vi "Calling or Specified VI's Clustered Controls Details, rev a.vi"(0 "Call heirarchy index\n(1 = calling VI, \n2 = its calling VI), etc)":i32=2, 11 "error in (no error)":errorcluster) -> (1 "Direct-access\ncontrols for\nrelabeling":refnum<vi>[](array[refnum]), 2 "Refs to controls on panel":refnum<vi>[](array[refnum]), 3 "Direct-access\ncontrols for\nrelabeling: captions":string[](array[string])=["Application Directory", "Direct Name 1", "Direct Position 1", "Direct Jog - 1", "Direct Jog + 1", "Direct Step (mm) 1", "Direct Halt Axis 1", "Direct Settings 1", "Direct Moving 1", "Direct New target 1", "Direct OK 1", "Direct Home Axis 1", "Direct Home Axis 2", "Direct OK 2", "Direct New target 2", "Direct Moving 2", "Direct Settings 2", "Direct Halt Axis 2", "Direct Step (mm) 2", "Direct Jog + 2", "Direct Jog - 2", "Direct Position 2", "Direct Name 2", "Direct Home Axis 3", "Direct OK 3", "Direct New target 3", "Direct Moving 3", "Direct Settings 3", "Direct Halt Axis 3", "Direct Step (mm) 3", "Direct Jog + 3", "Direct Jog - 3", "Direct Position 3", "Direct Name 3", "Direct Home Axis 4", "Direct OK 4", "Direct New target 4", "Direct Moving 4", "Direct Settings 4", "Direct Halt Axis 4", "Direct Step (mm) 4", "Direct Jog + 4", "Direct Jog - 4", "Direct Position 4", "Direct Name 4", "Direct Home Axis 5", "Direct OK 5", "Direct New target 5", "Direct Moving 5", "Direct Settings 5", "Direct Halt Axis 5", "Direct Step (mm) 5", "Direct Jog + 5", "Direct Jog - 5", "Direct Position 5", "Direct Name 5", "Direct Home Axis 6", "Direct OK 6", "Direct New target 6", "Direct Moving 6", "Direct Settings 6", "Direct Halt Axis 6", "Direct Step (mm) 6", "Direct Jog + 6", "Direct Jog - 6", "Direct Position 6", "Direct Name 6"], 4 "Names of Clusters":string[](array[string])=["error out"], 6 "Controls in\nthose clusters":string[][](array[string])=[["status", "code", "source"]], 10 "Refs to clusters":refnum<vi>[](array[refnum]), 12 "Controls directly on tab panes":string[](array[string])=["Interface", "S/N", "System no.", "Input XY bulls-eye", "Output XY bulls-eye", "Input Z bulls-eye", "RS Start", "RS Input XY:Enable", "RS Output XY:Enable", "RS Input XY:Status", "RS Output XY:Status", "RS Display Raw Data", "RS Input X:Range", "RS Input Y:Range", "RS Input Y:Step", "GS Start", "GS Display Raw Data", "I(t)", "Power Meter", "Output Z bulls-eye", "stop", "ID", "RS Frequency", "RS Input X:Center", "RS Input Y:Center", "RS Output X:Range", "RS Output Y:Range", "RS Output Y:Step", "RS Output X:Center", "RS Output Y:Center", "RS Input XY:Duration", "RS Output XY:Duration", "idle loop (msec)", "RS:Settle at 1st corner", "Axis role file", "Application Directory", "GS Status", "Power Meter Average", "RS Input XY:Swap Axes", "RS Output XY:Swap Axes", "PZT Input X:Position", "PZT Input Y:Position", "PZT Output X:Position", "PZT Output Y:Position", "PZT Input Z:Position", "PZT Output Z:Position", "RS Status", "PZT motion", "Motor motion", "Motor Input X:Name", "Motor Input X:Position", "Motor Input X:Jog +", "Motor Input X:Jog -", "Motor Input X:Step (mm)", "Motor Input X:Halt Axis", "Motor Input X:Settings", "Motor Input X:Moving", "Motor Input X:New Target", "Motor Input X:OK", "Motor Input X:Home Axis", "Motor Input Y:Home Axis", "Motor Input Y:OK", "Motor Input Y:New Target", "Motor Input Y:Moving", "Motor Input Y:Settings", "Motor Input Y:Halt Axis", "Motor Input Y:Step (mm)", "Motor Input Y:Jog -", "Motor Input Y:Jog +", "Motor Input Y:Position", "Motor Input Y:Name", "Motor Input Z:Home Axis", "Motor Input Z:OK", "Motor Input Z:New Target", "Motor Input Z:Moving", "Motor Input Z:Settings", "Motor Input Z:Halt Axis", "Motor Input Z:Step (mm)", "Motor Input Z:Jog -", "Motor Input Z:Jog +", "Motor Input Z:Position", "Motor Input Z:Name", "Motor Output X:Home Axis", "Motor Output X:OK", "Motor Output X:New Target", "Motor Output X:Moving", "Motor Output X:Settings", "Motor Output X:Halt Axis", "Motor Output X:Step (mm)", "Motor Output X:Jog -", "Motor Output X:Jog +", "Motor Output X:Position", "Motor Output X:Name", "Motor Output Y:Home Axis", "Motor Output Y:OK", "Motor Output Y:New Target", "Motor Output Y:Moving", "Motor Output Y:Settings", "Motor Output Y:Halt Axis", "Motor Output Y:Step (mm)", "Motor Output Y:Jog -", "Motor Output Y:Jog +", "Motor Output Y:Position", "Motor Output Y:Name", "Motor Output Z:Home Axis", "Motor Output Z:OK", "Motor Output Z:New Target", "Motor Output Z:Moving", "Motor Output Z:Settings", "Motor Output Z:Halt Axis", "Motor Output Z:Step (mm)", "Motor Output Z:Jog -", "Motor Output Z:Jog +", "Motor Output Z:Position", "Motor Output Z:Name", "GS Input XY:Enable", "GS Output XY:Enable", "GS Input Z:Enable", "GS Output Z:Enable", "GS Input XY:Status", "GS Output XY:Status", "GS Input Z:Status", "GS Output Z:Status", "RS Fit", "RS:Lower Clip Level", "RS:Upper Clip Level", "GS:Couple Processes", "FW", "RS Input:Successful", "GS Input XY:Success", "GS Output XY:Success", "GS Input Z:Success", "GS Output Z:Success", "RS Input:Threshold (mW)", "RS Output:Threshold (mW)", "RS Output:Successful", "Default settling window", "Scan axis center", "Step axis center", "Z axis center", "NxM Dithers", "RS Input XY:Data", "RS Output XY:Data", "error out", "Override Pane", "GS Input XY:Duration", "GS Output XY:Duration", "GS Input Z:Duration", "GS Input Z:Duration", "PZT Input X:New Target", "Scan Processes (from axis roles file)", "GS Parameters:Update", "PZT Input Y:New Target", "PZT Output X:New Target", "PZT Output Y:New Target", "PZT Output Z:New Target", "PZT Input Z:New Target", "GS Input XY:HZ", "GS Input XY:V", "GS Input XY:MDC", "GS Input XY:MINR", "GS Input XY:MAXR", "GS Input XY:ML", "GS Input XY:SP", "GS Output XY:HZ", "GS Output XY:V", "GS Output XY:MDC", "GS Output XY:MINR", "GS Output XY:MAXR", "GS Output XY:ML", "GS Output XY:SP", "GS Input Z:HZ", "GS Input Z:V", "GS Input Z:MDC", "GS Input Z:MINR", "GS Input Z:MAXR", "GS Input Z:ML", "GS Input Z:SP", "GS Output Z:HZ", "GS Output Z:V", "GS Output Z:MDC", "GS Output Z:MINR", "GS Output Z:MAXR", "GS Output Z:ML", "GS Output Z:SP", "GS Input XY process name", "GS Input XY StepAxNumber", "GS Input XY ScanAxNumber", "GS Input XY ScanAxName", "GS Input XY StepAxName", "GS Output XY process name", "GS Output XY StepAxNumber", "GS Output XY ScanAxNumber", "GS Output XY ScanAxName", "GS Output XY StepAxName", "GS Input Z process name", "GS Input Z StepAxNumber", "GS Input Z ScanAxNumber", "GS Input Z ScanAxName", "GS Input Z StepAxName", "GS Output Z process name", "GS Output Z StepAxNumber", "GS Output Z ScanAxNumber", "GS Output Z ScanAxName", "GS Output Z StepAxName", "msec timestamp"], 13 "Refs to controls directly on tab panes":refnum<vi>[](array[refnum]), 14 "Controls on panel":string[](array[string])=["Halt Homing", "Tab Control", "Names of Clusters", "Controls in clusters", "Refs to clusters", "PZT Input X:OK", "PZT Input Y:OK", "PZT Input Z:OK", "PZT Output X:OK", "PZT Output Y:OK", "PZT Output Z:OK"], 15 "error out":errorcluster)   [LabVIEW 2023]
panel:
  out "ref'd VI":string
  out "Array":string[](array[string])=["Array", "Array", "Array"]
  out "Arrays":string[](array[string])=["Names of Clusters", "Controls in clusters", "Refs to clusters"]
  out "Refs to arrays":refnum<vi>[](array[refnum])
  out "Names of TabControls":string[](array[string])=["Tab Control"]
  out "Refs to TabControls":refnum<vi>[](array[refnum])
  out "Types of Controls\non panel":string[](array[string])=["Boolean", "TabControl", "Array", "Array", "Array", "Boolean", "Boolean", "Boolean", "Boolean", "Boolean", "Boolean"]
  # "This subVI finds the controls that exist on the front panel of the calling VI (OR a \nspecified VI), then selects just-the-clusters from that list.  It then finds the elements of each cluster.\n\nIF the calling VI has tab controls, the structure of this VI must accommodate the number of pages for each tab control.  Here we have nine configurations: 2-10 pages.  Add to these as necessary to accommodate the configuration of the calling VI.\n\nThis VI does not handle calling VIs with tab controls containing tab controls containing clusters...\n\nSee further discussion in the block diagram."
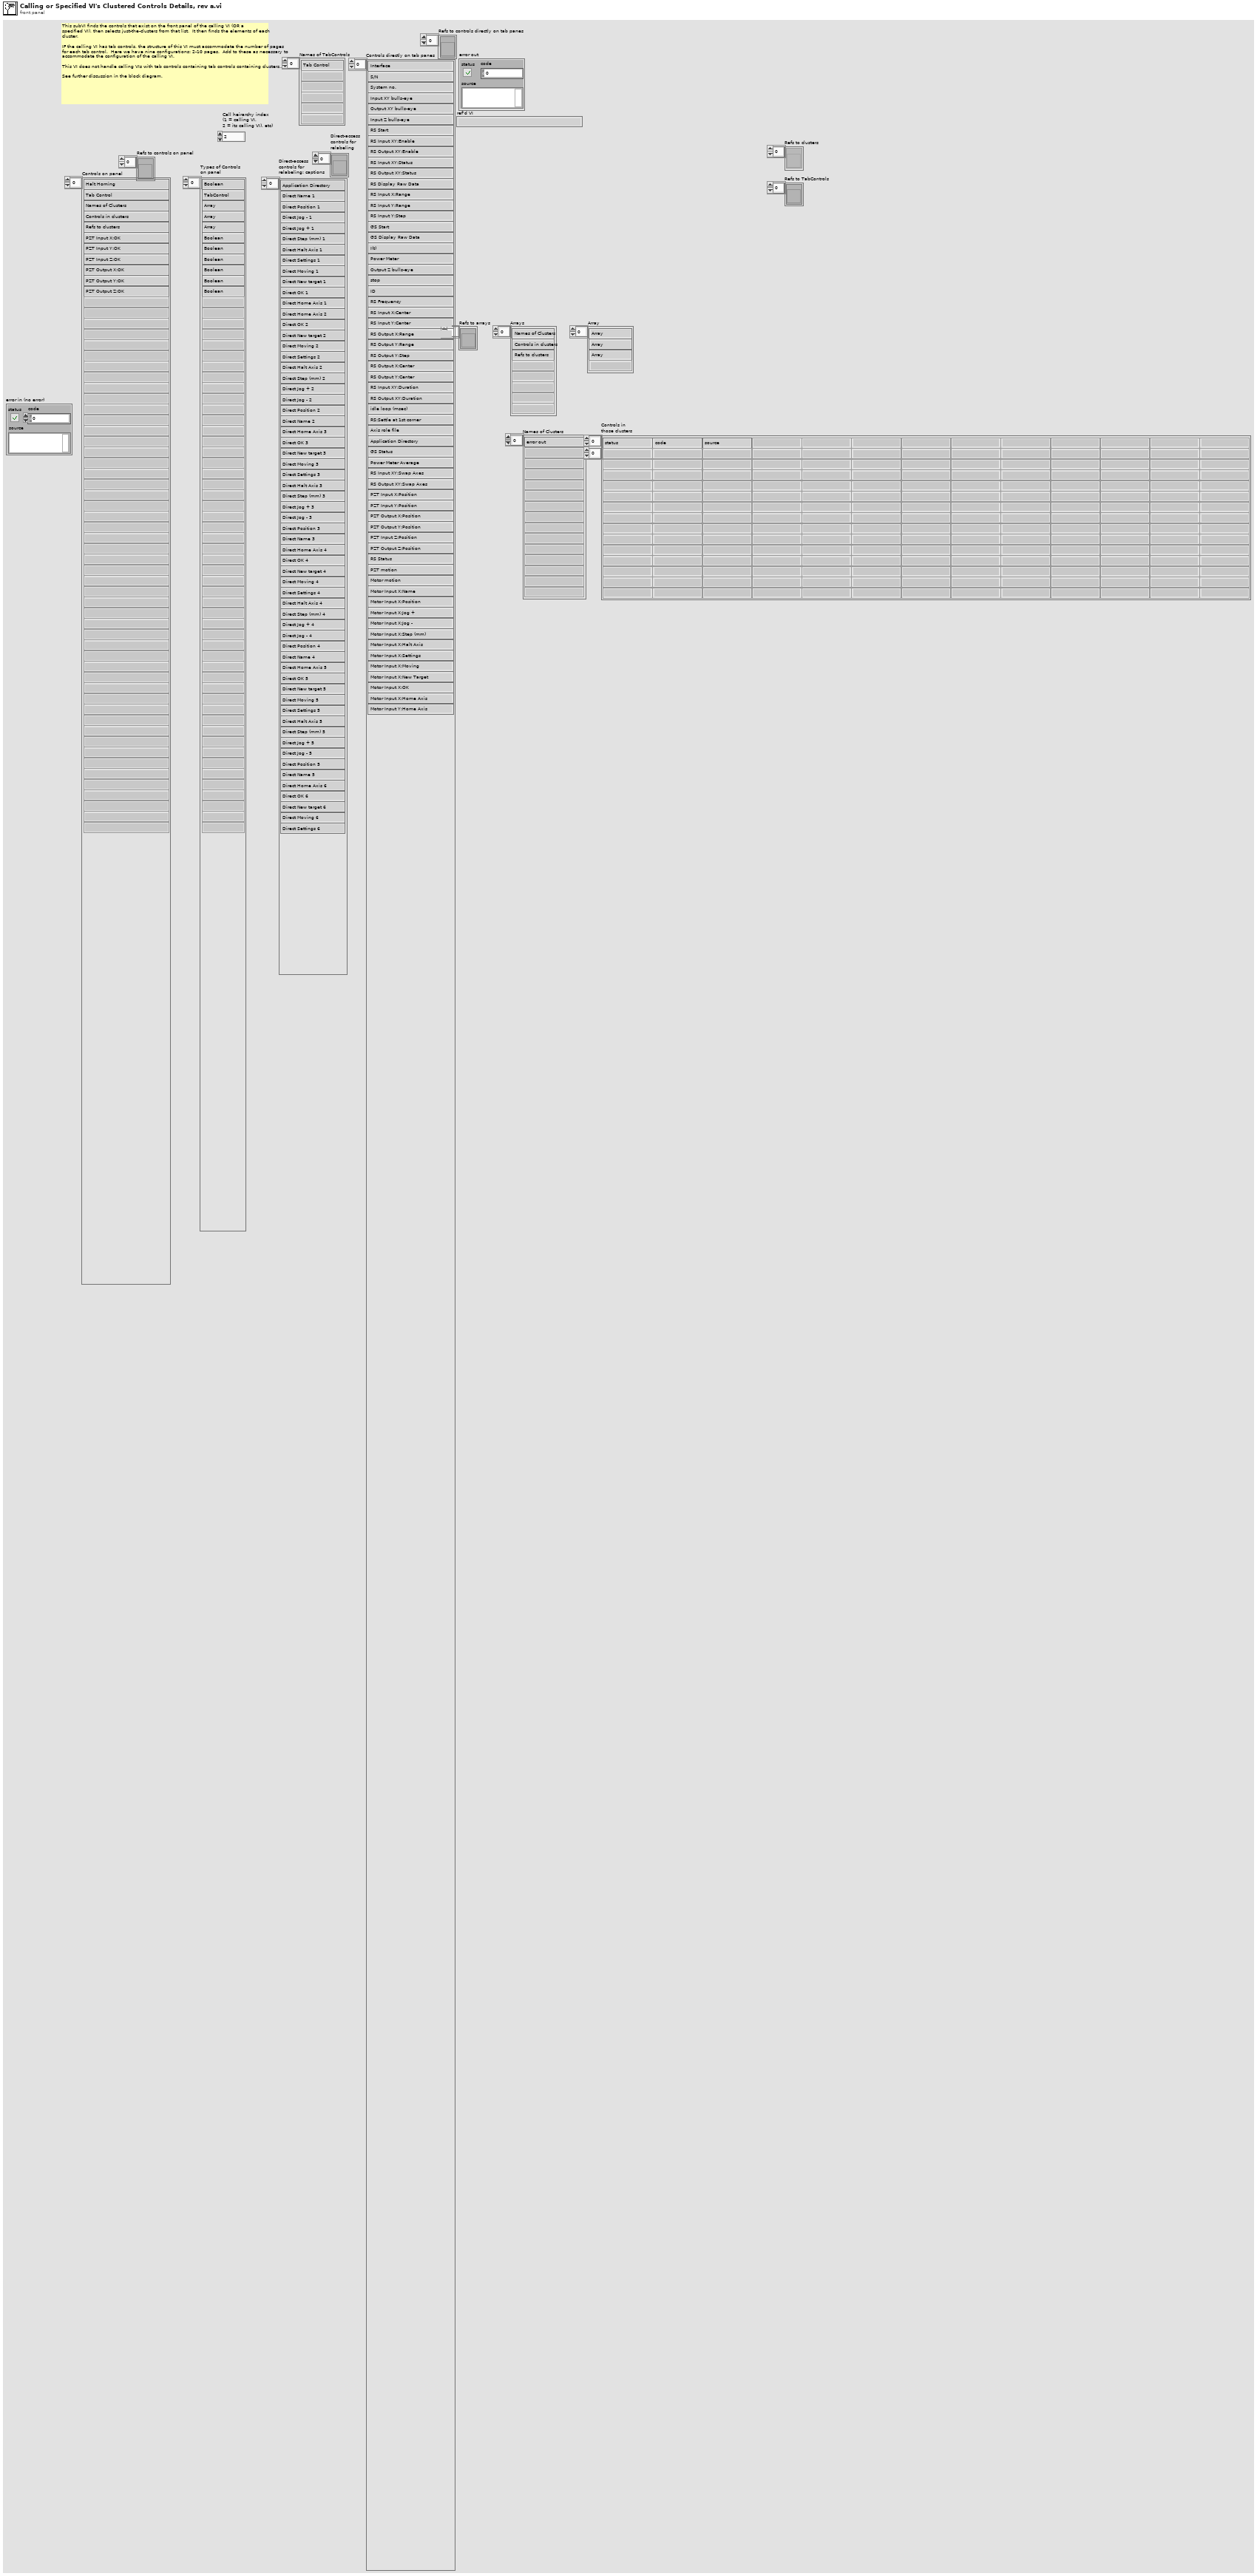
[diagram p1: front panel]
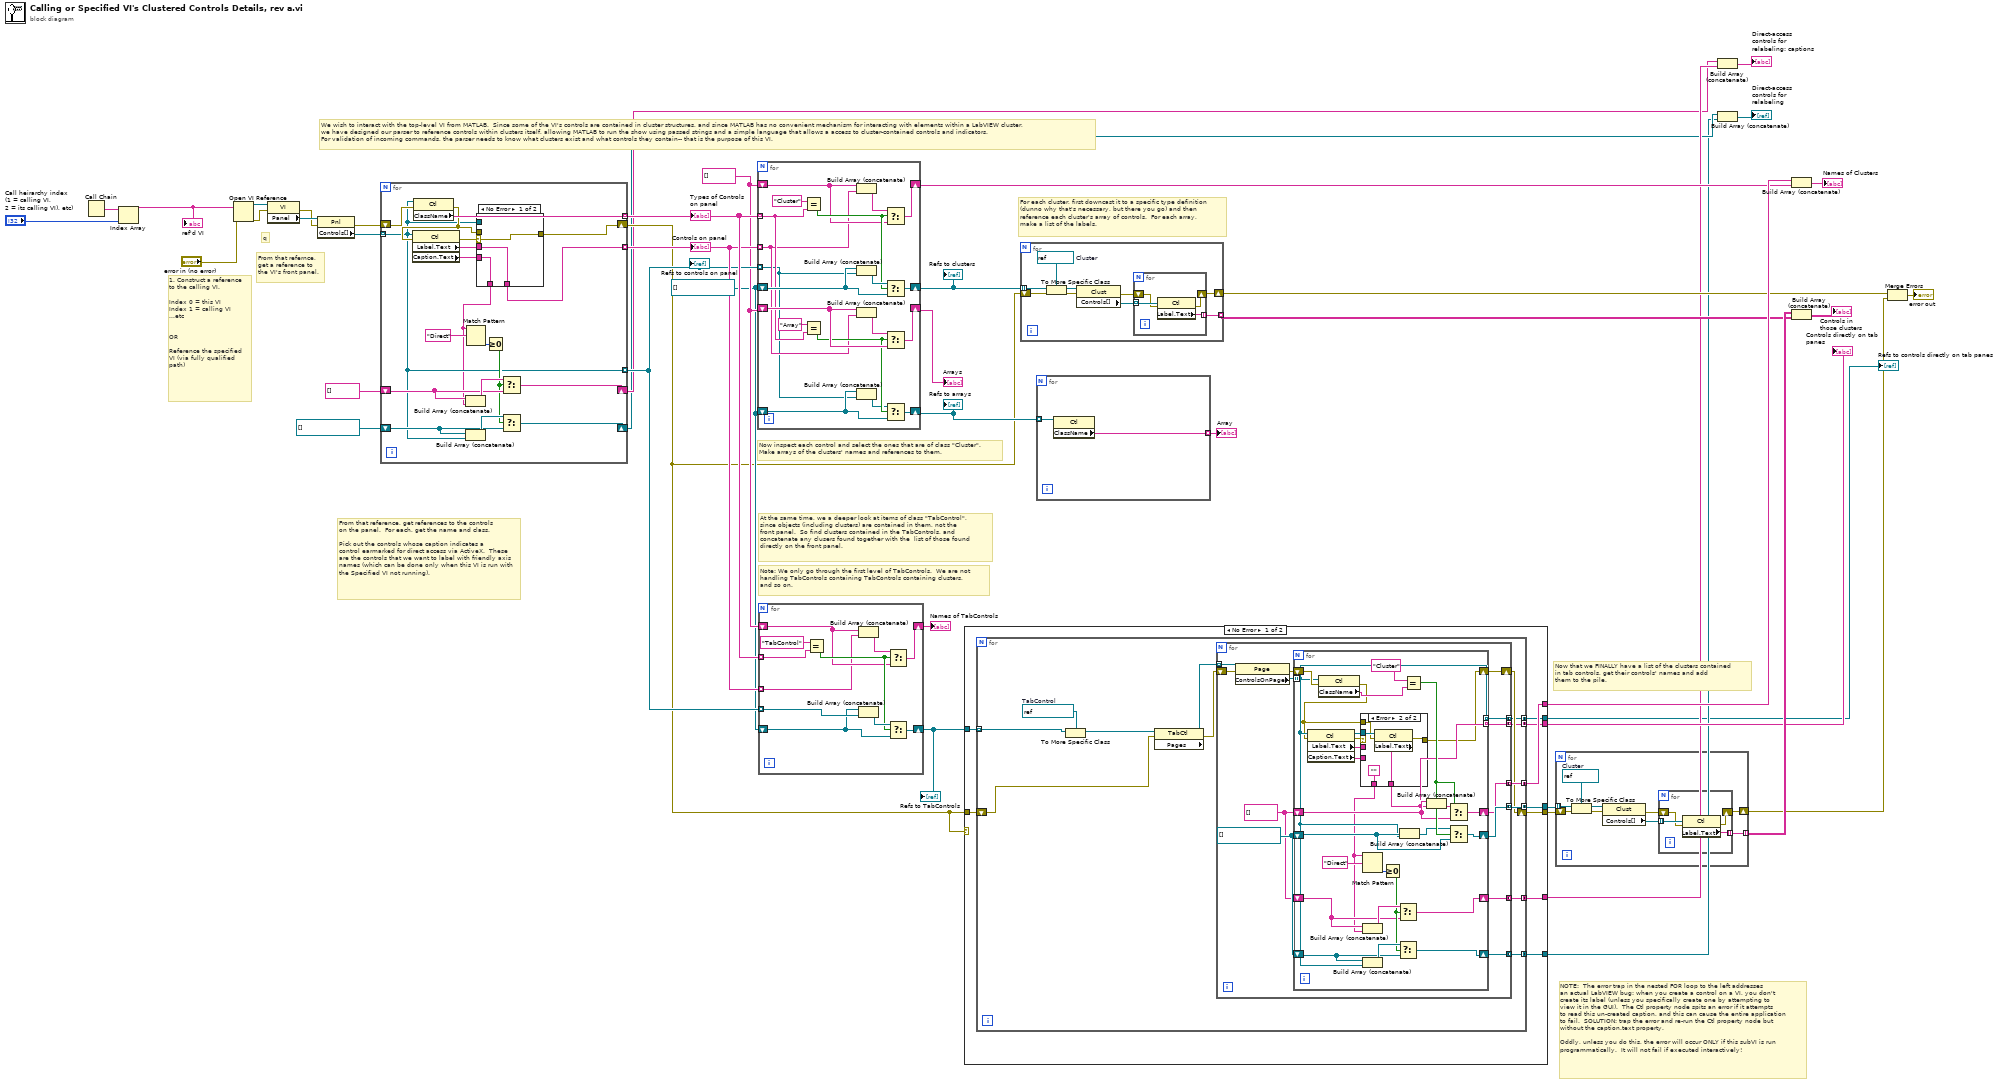
[diagram p0: block diagram]
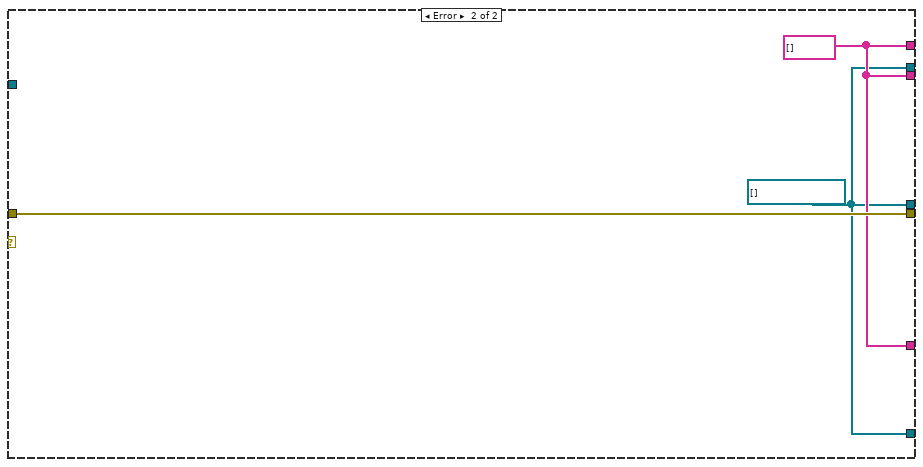
[diagram p3: hidden frame]
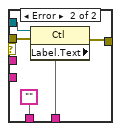
[diagram p4: hidden frame]
diagram:
  w17 = refnum<vi>[] []
  w18 = string[] []
  # "q"
  # "NOTE:  The error trap in the nested FOR loop to the left addresses\nan actual LabVIEW bug: when you create a control on a VI, you don't\ncreate its label (unless you specifically create one by attempting to \nview it in the GUI).  The Ctl property node spits an error if it attempts \nto read this un-created caption, and this can cause the entire application\nto fail.  SOLUTION: trap the error and re-run the Ctl property node but\nwithout the caption.text property.\n\nOddly, unless you do this, the error will occur ONLY if this subVI is run\nprogrammatically.  It will not fail if executed interactively!"
  # "We wish to interact with the top-level VI from MATLAB.  Since some of the VI's controls are contained in cluster structures, and since MATLAB has no convenient mechanism for interacting with elements within a LabVIEW cluster, \nwe have designed our parser to reference controls within clusters itself, allowing MATLAB to run the show using passed strings and a simple language that allows a access to cluster-contained controls and indicators.  \nFor validation of incoming commands, the parser needs to know what clusters exist and what controls they contain-- that is the purpose of this VI."
  # "Now that we FINALLY have a list of the clusters contained\nin tab controls, get their controls' names and add \nthem to the pile."
  # "Note: We only go through the first level of TabControls.  We are not\nhandling TabControls containing TabControls containing clusters,\nand so on."
  # "At the same time, we a deeper look at items of class \"TabControl\", \nsince objects (including clusters) are contained in them, not the\nfront panel.  So find clusters contained in the TabControls, and \nconcatenate any clusers found together with the  list of those found \ndirectly on the front panel."
  # "For each cluster, first downcast it to a specific type definition\n(dunno why that's necessary, but there you go) and then\nreference each cluster's array of controls.  For each array,\nmake a list of the labels."
  # "Now inspect each control and select the ones that are of class \"Cluster\".\nMake arrays of the clusters' names and references to them."
  # "From that reference, get references to the controls\non the panel.  For each, get the name and class.\n\nPick out the controls whose caption indicates a \ncontrol earmarked for direct access via ActiveX.  These are the controls that we want to label with friendly axis names (which can be done only when this VI is run with the Specified VI not running)."
  # "From that refernce,\nget a reference to\nthe VI's front panel."
  # "1. Construct a reference\nto the calling VI.  \n\nIndex 0 = this VI\nIndex 1 = calling VI\n...etc\n\n\nOR\n\nReference the specified\nVI (via fully qualified\npath)"
  n1 = Call Chain() -> (call chain=w40:string[])
  n2 = Index Array(array=w40, index="Call heirarchy index\n(1 = calling VI, \n2 = its calling VI), etc)") -> (element=w2:string)
  "ref'd VI" <- w2
  n3 = Open VI Reference(vi path=w2, error in (no error)="error in (no error)") -> (vi reference=w39:refnum<vi>, error out=w37:errorcluster)  [unwired: 4 in]
  n4 = property class="VI"(reference=w39, error in=w37) -> (error out=w36:errorcluster, "Panel"=w43:refnum<vi>)  [unwired: 1 out]
  n5 = property class="Pnl"(reference=w43, error in=w36) -> (error out=w35:errorcluster, "Controls[]"=w42:refnum<vi>[])  [unwired: 1 out]
  n6 = for {
    tunnel: w42 -> [w48] mode=indexing
    tunnel: [w45] -> w32 mode=indexing
    tunnel: [w62] -> w33 mode=indexing
    tunnel: [w48] -> w31 mode=indexing
    shift-right: [w50] -> w10
    shift-left: w35 -> [w61]
    shift-right: [w60] -> w8
    shift-left: string[] [] -> [w58]
    shift-right: [w56] -> w6
    shift-left: refnum<vi>[] [] -> [w55]
    n7 = property class="Ctl"(reference=w48, error in=w61) -> (error out=w49:errorcluster, "ClassName"=w62:string)  [unwired: 1 out]
    n8 = property class="Ctl"(reference=w48, error in=w49) -> (error out=w51:errorcluster, "Label.Text"=w47:string, "Caption.Text"=w46:string)  [unwired: 1 out]
    n9 = Build Array (concatenate)(w55, w48) -> (w57:refnum<vi>[])
    n10 = case shown="No Error" w51 {
      selector: w51 -> [w64 _]
      tunnel: w49 -> [_ w66]
      tunnel: w47 -> [w65 _]
      tunnel: [w65 w70] -> w45
      tunnel: w48 -> [_ w67]
      tunnel: [w64 w68] -> w50
      tunnel: [w63 ""] -> w44
      tunnel: w46 -> [w63 _]
      frame No Error {
      }
      frame Error {
        n11 = property class="Ctl"(reference=w67, error in=w66) -> (error out=w68:errorcluster, "Label.Text"=w70:string)  [unwired: 1 out]
      }
    }
    n12 = Build Array (concatenate)(w58, w44) -> (w59:string[])
    n13 = Match Pattern(string=w44, regular expression="Direct") -> (offset past match=w53:i32)  [unwired: 1 in, 3 out]
    n14 = Greater Or Equal To 0?(x=w53) -> (x >= 0?=w52:bool)
    n15 = Select(t=w59, s=w52, f=w58) -> (s? t:f=w60:string[])
    n16 = Select(t=w57, s=w52, f=w55) -> (s? t:f=w56:refnum<vi>[])
  }
  "Controls on panel" <- w32
  "Types of Controls\non panel" <- w33
  "Refs to controls on panel" <- w31
  n17 = for {
    tunnel: w33 -> [w74] mode=indexing
    tunnel: w32 -> [w73] mode=indexing
    shift-right: [w87] -> w25
    shift-left: w18 -> [w83]
    tunnel: w31 -> [w72] mode=indexing
    shift-right: [w85] -> w41
    shift-left: w17 -> [w82]
    shift-right: [w71] -> w16
    shift-left: w18 -> [w80]
    shift-right: [w78] -> w15
    shift-left: w17 -> [w81]
    n18 = Equal?(x="Cluster", y=w74) -> (x = y?=w84:bool)
    n19 = Equal?(x="Array", y=w74) -> (x = y?=w79:bool)
    n20 = Build Array (concatenate)(w83, w73) -> (w88:string[])
    n21 = Build Array (concatenate)(w82, w72) -> (w86:refnum<vi>[])
    n22 = Build Array (concatenate)(w80, w73) -> (w76:string[])
    n23 = Build Array (concatenate)(w81, w72) -> (w77:refnum<vi>[])
    n24 = Select(t=w88, s=w84, f=w83) -> (s? t:f=w87:string[])
    n25 = Select(t=w86, s=w84, f=w82) -> (s? t:f=w85:refnum<vi>[])
    n26 = Select(t=w76, s=w79, f=w80) -> (s? t:f=w71:string[])
    n27 = Select(t=w77, s=w79, f=w81) -> (s? t:f=w78:refnum<vi>[])
  }
  "Refs to clusters" <- w41
  "Refs to arrays" <- w15
  "Arrays" <- w16
  n28 = for {
    tunnel: w33 -> [w100] mode=indexing
    tunnel: w32 -> [w92] mode=indexing
    shift-right: [w97] -> w34
    shift-left: w18 -> [w93]
    tunnel: w31 -> [w91] mode=indexing
    shift-right: [w95] -> w30
    shift-left: w17 -> [w90]
    n29 = Equal?(x="TabControl", y=w100) -> (x = y?=w94:bool)
    n30 = Build Array (concatenate)(w93, w92) -> (w98:string[])
    n31 = Build Array (concatenate)(w90, w91) -> (w96:refnum<vi>[])
    n32 = Select(t=w98, s=w94, f=w93) -> (s? t:f=w97:string[])
    n33 = Select(t=w96, s=w94, f=w90) -> (s? t:f=w95:refnum<vi>[])
  }
  "Names of TabControls" <- w34
  "Refs to TabControls" <- w30
  n34 = case shown="No Error" w10 {
    tunnel: w30 -> [w109 _]
    tunnel: [w108 w172] -> w29
    tunnel: [w107 w173] -> w26
    tunnel: [w106 w174] -> w22
    tunnel: w10 -> [w105 w174]
    tunnel: [w104 w173] -> w13
    tunnel: [w103 w173] -> w9
    tunnel: [w102 w172] -> w5
    tunnel: [w101 w172] -> w3
    frame No Error {
      n35 = for {
        tunnel: w109 -> [w112] mode=indexing
        tunnel: [w121] -> w108 mode=concatenating
        tunnel: [w120] -> w107 mode=concatenating
        shift-right: [w118] -> w106
        shift-left: w105 -> [w113]
        tunnel: [w117] -> w104 mode=concatenating
        tunnel: [w116] -> w103 mode=concatenating
        tunnel: [w115] -> w102 mode=concatenating
        tunnel: [w114] -> w101 mode=concatenating
        w110 = refnum<vi> refnum  # TabControl
        n36 = To More Specific Class(target class=w110, reference=w112) -> (specific class reference=w111:refnum<vi>)  [unwired: 1 in, 1 out]
        n37 = property class="TabCtl"(reference=w111, error in=w113) -> (error out=w119:errorcluster, "Pages"=w122:refnum<vi>[])  [unwired: 1 out]
        n38 = for {
          tunnel: w122 -> [w135] mode=indexing
          tunnel: [w133] -> w121 mode=concatenating
          tunnel: [w132] -> w120 mode=concatenating
          shift-right: [w129] -> w118
          shift-left: w119 -> [w131]
          tunnel: [w128] -> w117 mode=concatenating
          tunnel: [w125] -> w116 mode=concatenating
          tunnel: [w124] -> w115 mode=concatenating
          tunnel: [w123] -> w114 mode=concatenating
          w126 = string[] []
          w127 = refnum<vi>[] []
          n39 = property class="Page"(reference=w135, error in=w131) -> (error out=w130:errorcluster, "ControlsOnPage"=w134:refnum<vi>[])  [unwired: 1 out]
          n40 = for {
            tunnel: w134 -> [w144] mode=indexing
            shift-right: [w160] -> w132
            shift-left: w126 -> [w156]
            shift-right: [w157] -> w133
            shift-left: w127 -> [w155]
            shift-right: [w138] -> w129
            shift-left: w130 -> [w154]
            tunnel: [w140] -> w128 mode=indexing
            shift-right: [w145] -> w124
            shift-left: w127 -> [w146]
            shift-right: [w147] -> w125
            shift-left: w126 -> [w148]
            tunnel: [w144] -> w123 mode=indexing
            n41 = property class="Ctl"(reference=w144, error in=w154) -> (error out=w139:errorcluster, "ClassName"=w162:string)  [unwired: 1 out]
            n42 = property class="Ctl"(reference=w144, error in=w139) -> (reference out=w142:refnum<vi>, error out=w143:errorcluster, "Label.Text"=w141:string, "Caption.Text"=w136:string)
            n43 = case shown="Error" w143 {
              selector: w143 -> [w165 _]
              tunnel: w142 -> [_ w171]
              tunnel: w141 -> [w166 _]
              tunnel: [w166 w169] -> w140
              tunnel: w139 -> [_ w170]
              tunnel: [w165 w167] -> w138
              tunnel: [w164 ""] -> w137
              tunnel: w136 -> [w164 _]
              frame No Error {
              }
              frame Error {
                n44 = property class="Ctl"(reference=w171, error in=w170) -> (error out=w167:errorcluster, "Label.Text"=w169:string)  [unwired: 1 out]
              }
            }
            n45 = Build Array (concatenate)(w148, w137) -> (w153:string[])
            n46 = Build Array (concatenate)(w146, w144) -> (w152:refnum<vi>[])
            n47 = Match Pattern(string=w137, regular expression="Direct") -> (offset past match=w150:i32)  [unwired: 1 in, 3 out]
            n48 = Greater Or Equal To 0?(x=w150) -> (x >= 0?=w149:bool)
            n49 = Select(t=w153, s=w149, f=w148) -> (s? t:f=w147:string[])
            n50 = Select(t=w152, s=w149, f=w146) -> (s? t:f=w145:refnum<vi>[])
            n51 = Build Array (concatenate)(w155, w144) -> (w158:refnum<vi>[])
            n52 = Equal?(x="Cluster", y=w162) -> (x = y?=w159:bool)
            n53 = Build Array (concatenate)(w156, w140) -> (w161:string[])
            n54 = Select(t=w161, s=w159, f=w156) -> (s? t:f=w160:string[])
            n55 = Select(t=w158, s=w159, f=w155) -> (s? t:f=w157:refnum<vi>[])
          }
        }
      }
    }
    frame Error {
      w173 = string[] []
      w172 = refnum<vi>[] []
    }
  }
  "Controls directly on tab panes" <- w13
  "Refs to controls directly on tab panes" <- w3
  n56 = for {
    tunnel: w41 -> [w183] mode=indexing
    tunnel: [w179] -> w23 mode=indexing
    shift-right: [w175] -> w20
    shift-left: w10 -> [w178]
    w182 = refnum<vi> refnum  # Cluster
    n57 = To More Specific Class(target class=w182, reference=w183, error in=w178) -> (specific class reference=w181:refnum<vi>, error out=w177:errorcluster)
    n58 = property class="Clust"(reference=w181, error in=w177) -> (error out=w176:errorcluster, "Controls[]"=w180:refnum<vi>[])  [unwired: 1 out]
    n59 = for {
      tunnel: w180 -> [w187] mode=indexing
      tunnel: [w186] -> w179 mode=indexing
      shift-right: [w184] -> w175
      shift-left: w176 -> [w185]
      n60 = property class="Ctl"(reference=w187, error in=w185) -> (error out=w184:errorcluster, "Label.Text"=w186:string)  [unwired: 1 out]
    }
  }
  n61 = for {
    tunnel: w15 -> [w189] mode=indexing
    tunnel: [w188] -> w14 mode=indexing
    n62 = property class="Ctl"(reference=w189) -> ("ClassName"=w188:string)  [unwired: 1 in, 2 out]
  }
  "Array" <- w14
  n63 = for {
    tunnel: w29 -> [w198] mode=indexing
    tunnel: [w194] -> w24 mode=indexing
    shift-right: [w190] -> w19
    shift-left: w22 -> [w193]
    w197 = refnum<vi> refnum  # Cluster
    n64 = To More Specific Class(target class=w197, reference=w198, error in=w193) -> (specific class reference=w196:refnum<vi>, error out=w192:errorcluster)
    n65 = property class="Clust"(reference=w196, error in=w192) -> (error out=w191:errorcluster, "Controls[]"=w195:refnum<vi>[])  [unwired: 1 out]
    n66 = for {
      tunnel: w195 -> [w202] mode=indexing
      tunnel: [w201] -> w194 mode=indexing
      shift-right: [w199] -> w190
      shift-left: w191 -> [w200]
      n67 = property class="Ctl"(reference=w202, error in=w200) -> (error out=w199:errorcluster, "Label.Text"=w201:string)  [unwired: 1 out]
    }
  }
  n68 = Build Array (concatenate)(w8, w9) -> (→"Direct-access\ncontrols for\nrelabeling: captions":string[])
  n69 = Build Array (concatenate)(w6, w5) -> (→"Direct-access\ncontrols for\nrelabeling":refnum<vi>[])
  n70 = Build Array (concatenate)(w26, w25) -> (→"Names of Clusters":string[])
  n71 = Build Array (concatenate)(w24, w23) -> (→"Controls in\nthose clusters":string[][])
  n72 = Merge Errors(w20, w19) -> (→"error out":errorcluster)
